vi "Global VI for Localized Text.vi"() -> ()   [LabVIEW 2020, in "TdmsFileViewer.lvlib"]
uses:
  TdmsFileViewer.lvlib
panel:
  in  "False":string="false"
  in  "True":string="true"
  in  "pattern label tdms":string="TDMS File"
  in  "prompt tdms":string="Select a TDMS File"
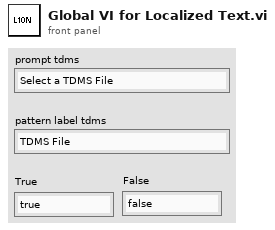
[diagram p1: front panel]
diagram:
